vi "Connect to Chassis by IP Address or Hostname.vi"(0 "session in":refnum<k21>, 1 "username":string, 2 "password":string, 5 "chassis IP address/hostname":string, 11 "error in (no error)":errorcluster, 12 "connect timeout (60 sec)":dbl=60.0) -> (4 "session out":refnum<k21>, 6 "chassis out":refnum<k21>, 15 "error out":errorcluster)   [LabVIEW 2020, in "SLSC.lvlib"]
doc: "Opens a network connection for a chassis by IP address or hostname. This VI shares network connections to the same chassis. If you cannot find the chassis via mDNS, ensure that the chassis is in the local configuration file. If the connect timeout expires before a connection is successfully established, this VI returns an error."
uses:
  <vilib>/SLSC/SLSC.lvlib
  nislsclvapi.dll
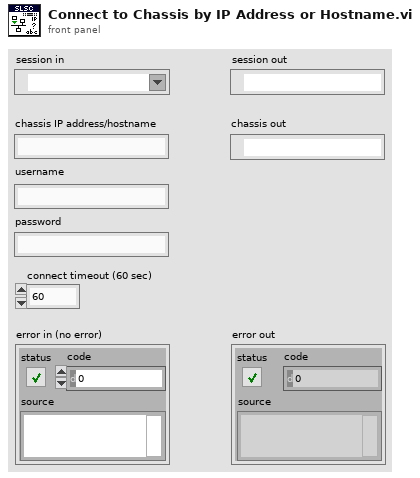
[diagram p1: front panel]
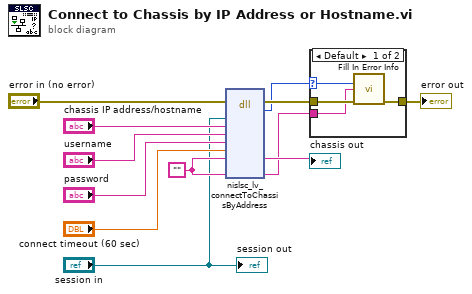
[diagram p0: block diagram]
diagram:
  w7 = ""
  n1 = dll-call lib="nislsclvapi.*" fn="nislsc_lv_connectToChassisByAddress"(error in="error in (no error)", "session"="session in", "address"="chassis IP address/hostname", "username"="username", "password"="password", "connectTimeout"="connect timeout (60 sec)", "chassis"=w7, "extendedErrorInfo"=w7) -> (error out=w5:errorcluster, "return type"=w1:i32, "chassis"=→"chassis out":string, "extendedErrorInfo"=w4:string)  [unwired: 9 in, 1 out]
  n2 = case shown="Default" w1 {
    selector: w1 -> [w14 _]
    tunnel: w4 -> [w15 _]
    tunnel: w5 -> [w16 w17]
    tunnel: [w13 w17] -> w3
    frame Default {
      n3 = call <vilib>:"Fill In Error Info.vi"("status code"=w14, "extended error info"=w15, "error in"=w16) -> ("error out"=w13:errorcluster)  [unwired: 12 in]
    }
    frame 0 {
    }
  }
  "error out" <- w3
  "session out" <- "session in"
